vi "PID Arm Range.vi"(1 "Input PID":dbl) -> (0 "Output Range":dbl)   [LabVIEW 2017]
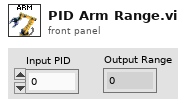
[diagram p1: front panel]
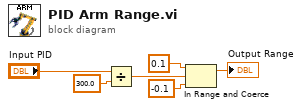
[diagram p0: block diagram]
diagram:
  n1 = Divide(x="Input PID", y=300.0) -> (x/y=w4:dbl)
  n2 = In Range and Coerce(upper limit=0.1, x=w4, lower limit=-0.1) -> (coerced(x)=→"Output Range":dbl)  [unwired: 1 out]
